vi "AlliGator Get Gate Image Series Folders.vi"(8 "Error In":errorcluster, 9 "pattern":string, 11 "Path":path) -> (0 "Error Out":errorcluster, 1 "Message":string, 2 "Timestamps":dbl[](array[numeric]), 3 "Time-Series Paths":path[](array[path]))   [LabVIEW 2021, in "AlliGator Files.lvlib"]
doc: "Reads valid folders of image in a time series."
uses:
  AlliGator Files.lvlib
  <userlib>/_OpenG.lib/array/array.llb/Filter 1D Array with Scalar (DBL)__ogtk.vi
  Strings/Strings.lvlib
  Scripts/AlliGator Scripts.lvlib
  Sound/Sound.lvlib
  <userlib>/_OpenG.lib/array/array.llb/openg_array.lvlib
panel:
  # "see the AlliGator License on the block diagram (Ctrl+E or Window:Show Block Diagram)"
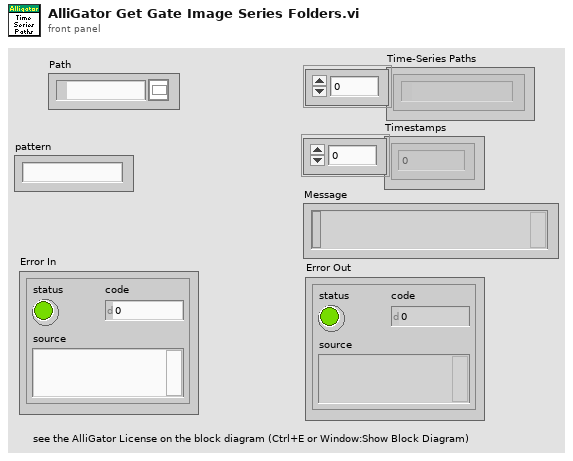
[diagram p1: front panel]
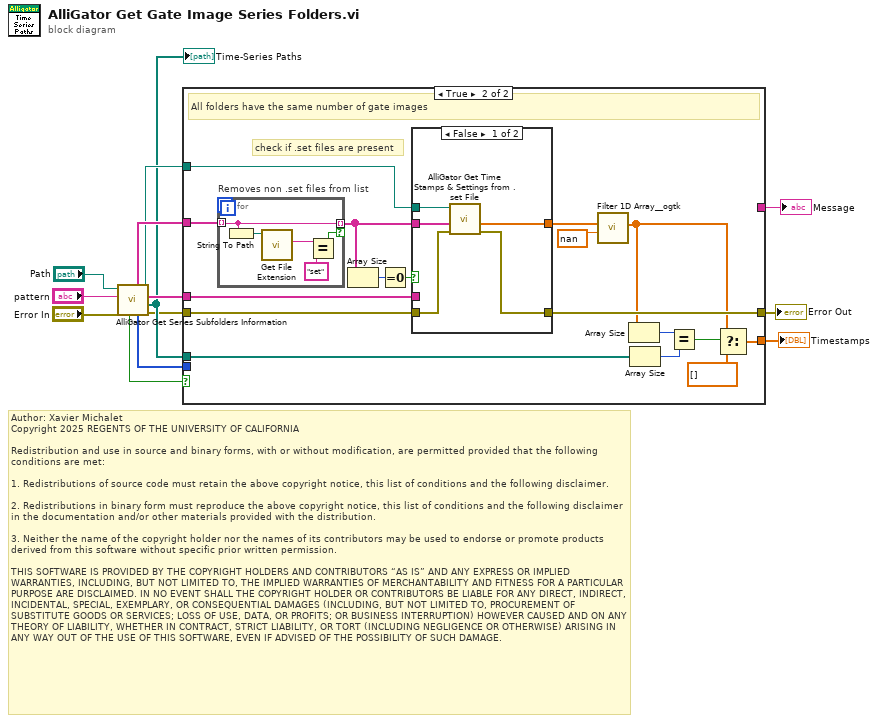
[diagram p0: block diagram]
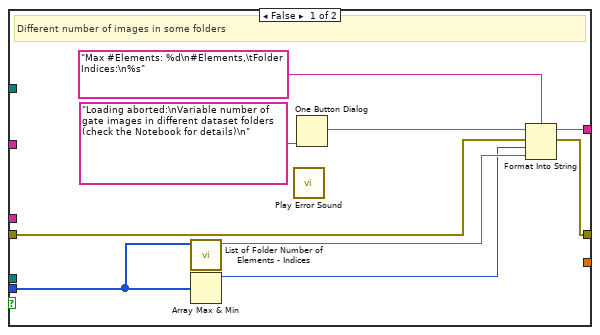
[diagram p2: hidden frame]
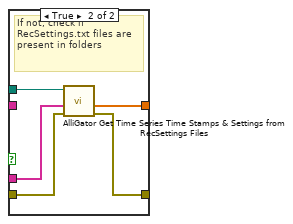
[diagram p3: hidden frame]
diagram:
  # "Author: Xavier Michalet\nCopyright 2025 REGENTS OF THE UNIVERSITY OF CALIFORNIA\n\nRedistribution and use in source and binary forms, with or without modification, are permitted provided that the following conditions are met:\n\n1. Redistributions of source code must retain the above copyright notice, this list of conditions and the following disclaimer.\n\n2. Redistributions in binary form must reproduce the above copyright notice, this list of conditions and the following disclaimer in the documentation and/or other materials provided with the distribution.\n\n3. Neither the name of the copyright holder nor the names of its contributors may be used to endorse or promote products derived from this software without specific prior written permission.\n\nTHIS SOFTWARE IS PROVIDED BY THE COPYRIGHT HOLDERS AND CONTRIBUTORS “AS IS” AND ANY EXPRESS OR IMPLIED WARRANTIES, INCLUDING, BUT NOT LIMITED TO, THE IMPLIED WARRANTIES OF MERCHANTABILITY AND FITNESS FOR A PARTICULAR PURPOSE ARE DISCLAIMED. IN NO EVENT SHALL THE COPYRIGHT HOLDER OR CONTRIBUTORS BE LIABLE FOR ANY DIRECT, INDIRECT, INCIDENTAL, SPECIAL, EXEMPLARY, OR CONSEQUENTIAL DAMAGES (INCLUDING, BUT NOT LIMITED TO, PROCUREMENT OF SUBSTITUTE GOODS OR SERVICES; LOSS OF USE, DATA, OR PROFITS; OR BUSINESS INTERRUPTION) HOWEVER CAUSED AND ON ANY THEORY OF LIABILITY, WHETHER IN CONTRACT, STRICT LIABILITY, OR TORT (INCLUDING NEGLIGENCE OR OTHERWISE) ARISING IN ANY WAY OUT OF THE USE OF THIS SOFTWARE, EVEN IF ADVISED OF THE POSSIBILITY OF SUCH DAMAGE."
  n1 = call "AlliGator Get Series Subfolders Information.vi"("error in (no error)"="Error In", "pattern"="pattern", "Path"="Path") -> ("error out"=w4:errorcluster, "Subfolder Paths"=w6:path[], "Sorted Subfolder Names"=w7:string[], "dup directory path"=w8:path, "# Files"=w1:i32[], "Files in the Root Folder"=w9:string[], "Same # Files?"=w2:bool)  [unwired: 2 in]
  "Time-Series Paths" <- w6
  n2 = case shown="True" w2 {
    tunnel: [w14 w25] -> w13
    tunnel: w8 -> [_ w27]
    tunnel: [w18 _] -> w12
    tunnel: w6 -> [_ w38]
    tunnel: [_ w34] -> w11
    tunnel: w9 -> [_ w32]
    tunnel: w4 -> [w15 w26]
    tunnel: w7 -> [_ w28]
    tunnel: w1 -> [w16 _]
    frame False {
      w21 = "Loading aborted:\nVariable number of gate images in different dataset folders (check the Notebook for details)\n" ("message")
      # "Different number of images in some folders"
      n3 = call "List of Folder Number of Elements - Indices.vi"("# Elements Array"=w16) -> ("Output String"=w19:string)  [unwired: 10 in]
      n4 = Array Max & Min(array=w16) -> (max value=w17:i32)  [unwired: 3 out]
      n5 = call "Play Error Sound.vi"() -> ()  [unwired: 27 in, 1 out]
      n6 = One Button Dialog(message=w21) -> ()  [unwired: 1 in, 1 out]
      n7 = Format Into String(format string="Max #Elements: %d\n#Elements,\tFolder Indices:\n%s", initial string=w21, error in=w15, w17, w19) -> (resulting string=w18:string, error out=w14:errorcluster)
    }
    frame True {
      # "check if .set files are present"
      # "All folders have the same number of gate images"
      n8 = for "Removes non .set files from list" {
        tunnel: w32 -> [w50] mode=indexing
        tunnel: [w50] -> w31 mode=indexing if=w49
        n9 = String To Path(string=w50) -> (path=w53:path)
        n10 = call <vilib>:"Get File Extension.vi"("file"=w53) -> ("lowercase file extension"=w52:string)  [unwired: 6 in, 4 out]
        n11 = Equal?(x=w52, y="set") -> (x = y?=w49:bool)
      }
      n12 = Array Size(array=w31) -> (size(s)=w30:i32)
      n13 = Equal To 0?(x=w30) -> (x = 0?=w29:bool)
      n14 = case shown="False" w29 {
        tunnel: w27 -> [w43 w48]
        tunnel: w31 -> [w42 _]
        tunnel: [w41 w46] -> w22
        tunnel: w28 -> [_ w47]
        tunnel: w26 -> [w40 w45]
        tunnel: [w39 w44] -> w25
        frame False {
          n15 = call "AlliGator Get Time Stamps & Settings from .set File.vi"("Error In"=w40, ".set File Names"=w42, "Folder Path"=w43) -> ("Error Out"=w39:errorcluster, "Time Stamps"=w41:dbl[])  [unwired: 6 in, 1 out]
        }
        frame True {
          # "If not, check if RecSettings.txt files are present in folders"
          n16 = call "AlliGator Get Time Series Time Stamps & Settings from RecSettings Files.vi"("Error In"=w45, "Sorted Folder Names"=w47, "Folder Path"=w48) -> ("Error Out"=w44:errorcluster, "Time Stamps"=w46:dbl[])  [unwired: 6 in, 1 out]
        }
      }
      n17 = call-poly <userlib>:"Filter 1D Array__ogtk.vi"("items to filter"=nan ("Time Stamp"), "array"=w22) -> ("filtered array"=w23:dbl[])  [unwired: 4 in, 1 out]
      n18 = Array Size(array=w23) -> (size(s)=w37:i32)
      n19 = Array Size(array=w38) -> (size(s)=w36:i32)
      n20 = Equal?(x=w37, y=w36) -> (x = y?=w35:bool)
      n21 = Select(t=w23, s=w35, f=dbl[] []) -> (s? t:f=w34:dbl[])
    }
  }
  "Error Out" <- w13
  "Message" <- w12
  "Timestamps" <- w11
